vi "buffer error.vi"(0 "Serial port asssistant model in":refnum<class "Serial port assistant model.lvclass">, 11 "error in (no error)":errorcluster) -> (4 "Serial port asssistant model out":refnum<class "Serial port assistant model.lvclass">, 15 "error out":errorcluster)   [LabVIEW 2022 SP3]
uses:
  Serial port assistant model.lvclass
  changed data--type.ctl
  Serial port assistant model.lvclass/Serial port assistant model.ctl
  C:/Users/ZSJ/Documents/Project/MV Plugin Architecture/Abstract Model/Abstract Model.lvlibp/Abstract Model.lvclass
  C:/Users/ZSJ/Documents/Project/MV Plugin Architecture/Demo/Model/Serial port assistant model.lvclass
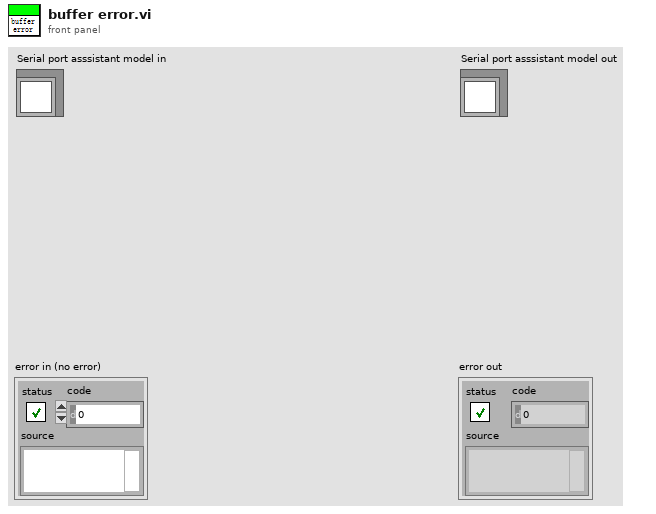
[diagram p1: front panel]
types:
  T1 = cluster{"changed data":string, "status":bool, "code":i32, "source":string}
  T2 = typedef "Serial port assistant model.lvlib/Serial port assistant model.lvclass/changed data--type.ctl" = cluster{"changed data":string}
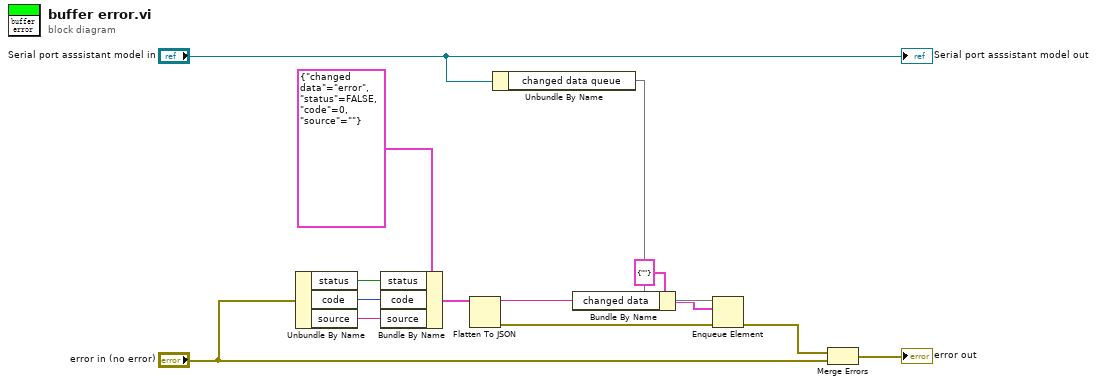
[diagram p0: block diagram]
diagram:
  n1 = Unbundle By Name("error in (no error)") -> ("status"=w8:bool, "code"=w7:i32, "source"=w6:string)
  n2 = Bundle By Name(cluster=T1 {"changed data"="error", "status"=FALSE, "code"=0, "source"=""}, "status"=w8, "code"=w7, "source"=w6) -> (w5:T1)
  n3 = Flatten To JSON(anything=w5) -> (JSON string=w4:string, 11:w10:errorcluster)  [unwired: 2 in]
  n4 = Unbundle By Name("Serial port asssistant model in") -> ("changed data queue"=w14)
  n5 = Bundle By Name(cluster=T2 {"changed data"=""} ("element"), "changed data"=w4) -> (w12:T2)
  n6 = Enqueue Element(queue=w14, element=w12, error in (no error)=w10) -> (error out=w3:errorcluster)  [unwired: 1 in, 2 out]
  n7 = Merge Errors(w3, "error in (no error)") -> (→"error out":errorcluster)
  "Serial port asssistant model out" <- "Serial port asssistant model in"
